vi "inout.vi"(8 "Step [mA]":dbl=25.0, 9 "Initial Value [mA]":dbl=250.0, 11 "# Steps":dbl=13.0) -> (0 "Array":dbl[](array[numeric]))   [LabVIEW 2021]
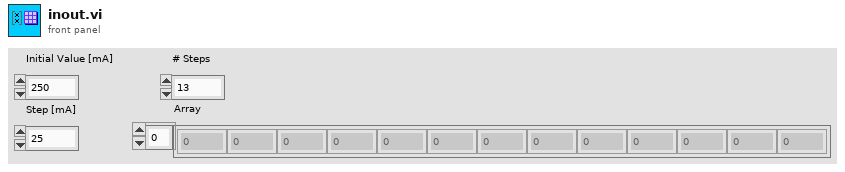
[diagram p1: front panel]
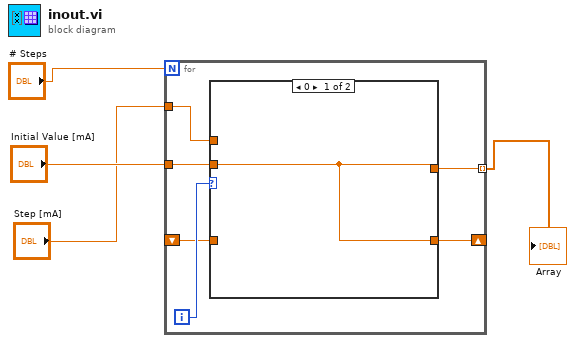
[diagram p0: block diagram]
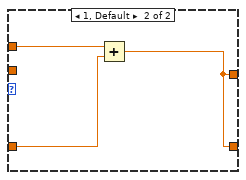
[diagram p2: hidden frame]
diagram:
  n1 = for {
    N: "# Steps" -> [_]
    tunnel: "Initial Value [mA]" -> [w9]
    tunnel: [w8] -> w1 mode=indexing
    tunnel: "Step [mA]" -> [w7]
    shift-right: [w6] -> _
    shift-left: _ -> [w5]
    i -> [w10]
    n2 = case shown="0" w10 {
      tunnel: [w11 w12] -> w8
      tunnel: w9 -> [w11 _]
      tunnel: w7 -> [_ w14]
      tunnel: [w11 w12] -> w6
      tunnel: w5 -> [_ w13]
      frame 0 {
      }
      frame 1, Default {
        n3 = Add(x=w14, y=w13) -> (x+y=w12:dbl)
      }
    }
  }
  "Array" <- w1
